vi "Read.vi"(8 "error in":errorcluster) -> (0 "error out":errorcluster)   [LabVIEW 2018, in "PC UDP Reader.lvlib"]
doc: "This subVI enqueues the named action in to the communications queue along with the input data."
uses:
  PC UDP Reader.lvlib
  Private Controls/Module Data.ctl
  Private Controls/Module Action.ctl
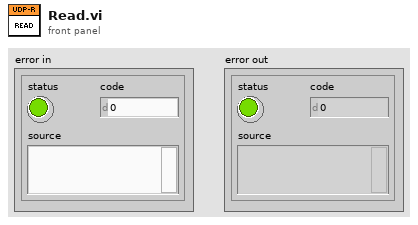
[diagram p1: front panel]
types:
  T1 = typedef "PC UDP Reader.lvlib/Module Data.ctl" = cluster{"Data":variant, "Action":T2}
  T2 = typedef "PC UDP Reader.lvlib/Module Action.ctl" = enum8{"Init", "Read", "Error", "Exit"}
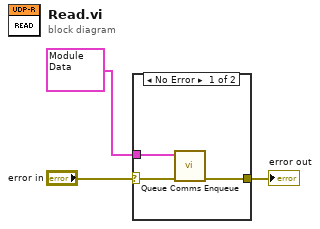
[diagram p0: block diagram]
diagram:
  n1 = case shown="No Error" "error in" {
    selector: "error in" -> [w5 w7]
    tunnel: [w6 w7] -> w3
    tunnel: T1 {"Data"=variant, "Action"=enum."Read"} ("element") -> [w4 _]
    frame No Error {
      n2 = call "Queue Comms Enqueue.vi"("error in (no error)"=w5, "element"=w4) -> ("error out"=w6:errorcluster)  [unwired: 9 in]
    }
    frame Error {
    }
  }
  "error out" <- w3
